vi "removeNode.vi"(0 "reference":refnum<class "AbstractNode.lvclass">, 1 "graph":refnum<class "Graph.lvclass">, 2 "node":refnum<class "AbstractNode.lvclass">, 5 "error in (no error)":errorcluster) -> (14 "reference out":refnum<class "AbstractNode.lvclass">, 19 "error out":errorcluster)   [LabVIEW 2020, in "AbstractNode.lvclass"]
uses:
  <resource>/Framework/Providers/Open_GDS/UML/AbstractNode_class/AbstractNode.lvclass
  <resource>/Framework/Providers/Open_GDS/UML/Graph_class/Graph.lvclass
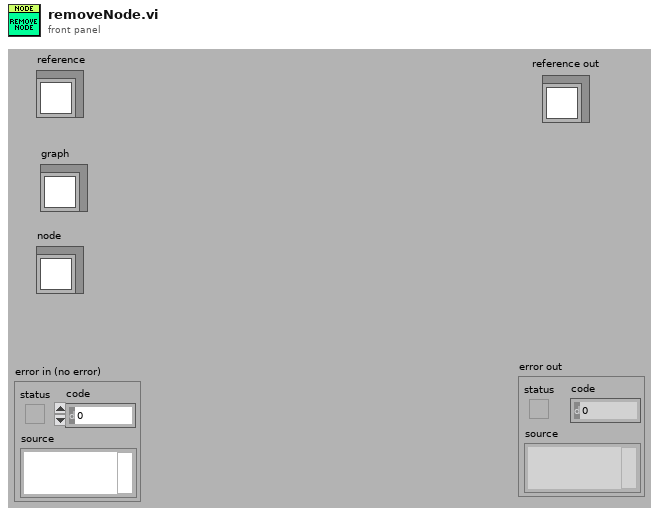
[diagram p1: front panel]
types:
  T1 = typedef "AbstractNode.lvclass/ObjectAttributes.ctl" = cluster{"parent":refnum<class "AbstractNode.lvclass">, "children":refnum<class "AbstractNode.lvclass">[], "Hidden":bool}
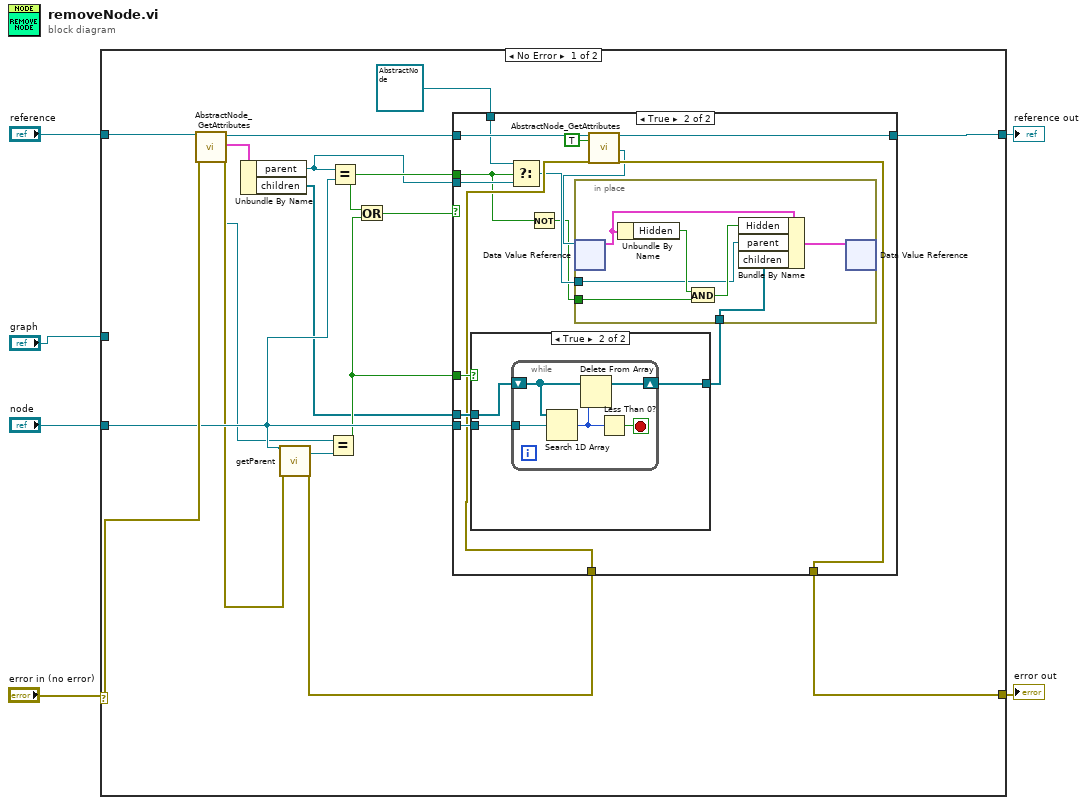
[diagram p0: block diagram]
diagram:
  n1 = case shown="No Error" "error in (no error)" {
    selector: "error in (no error)" -> [w19 w56]
    tunnel: "reference" -> [w22 w57]
    tunnel: [w21 w56] -> w5
    tunnel: [w20 w57] -> w4
    tunnel: "graph" -> [_ _]
    tunnel: "node" -> [w18 _]
    frame No Error {
      n2 = call <resource>:"AbstractNode_GetAttributes.vi"("reference in"=w22, "error in (no error)"=w19) -> ("reference out"=w9:refnum<class "AbstractNode.lvclass">, "Data"=w7:T1, "error out"=w13:errorcluster)  [unwired: 1 in, 14 out]
      n3 = Unbundle By Name(w7) -> ("parent"=w15:refnum<class "AbstractNode.lvclass">, "children"=w10:refnum<class "AbstractNode.lvclass">[])
      n4 = call-dynamic "getParent.vi"("reference"=w18, "error in (no error)"=w13) -> ("parentNode"=w12:refnum<class "AbstractNode.lvclass">, "error out"=w14:errorcluster)  [unwired: 13 in, 3 out]
      n5 = Equal?(x=w9, y=w12) -> (x = y?=w11:bool)
      n6 = Equal?(x=w15, y=w18) -> (x = y?=w16:bool)
      n7 = Or(x=w16, y=w11) -> (x .or. y?=w17:bool)
      n8 = case shown="True" w17 {
        tunnel: w9 -> [w24 w39]
        tunnel: [w24 w38] -> w20
        tunnel: w16 -> [_ w30]
        tunnel: w15 -> [_ w31]
        tunnel: w18 -> [_ w37]
        tunnel: w14 -> [w23 w33]
        tunnel: [w23 w36] -> w21
        tunnel: w11 -> [_ w35]
        tunnel: w10 -> [_ w34]
        tunnel: refnum<class "AbstractNode.lvclass"> refnum ("parent") -> [_ w32]
        frame False {
        }
        frame True {
          n9 = case shown="True" w35 {
            tunnel: w37 -> [_ w50]
            tunnel: w34 -> [w47 w49]
            tunnel: [w47 w48] -> w26
            frame False {
            }
            frame True {
              n10 = while {
                tunnel: w50 -> [w55]
                shift-right: [w53] -> w48
                shift-left: w49 -> [w54]
                stop <- w51 stop-if-true
                n11 = Search 1D Array(1D array=w54, element=w55) -> (index of element=w52:i32)  [unwired: 1 out]
                n12 = Delete From Array(array=w54, index=w52) -> (array with subset deleted=w53:refnum<class "AbstractNode.lvclass">[])  [unwired: 1 in, 1 out]
                n13 = Less Than 0?(x=w52) -> (x < 0?=w51:bool)
              }
            }
          }
          n14 = Select(t=w32, s=w30, f=w31) -> (s? t:f=w27:refnum<class "AbstractNode.lvclass">)
          n15 = Not(x=w30) -> (.not. x?=w25:bool)
          n16 = call <resource>:"AbstractNode_GetAttributes.vi"("reference in"=w39, "OnlyGetDvrReference(False)"=TRUE, "error in (no error)"=w33) -> ("reference out"=w38:refnum<class "AbstractNode.lvclass">, "DataRef"=w28:refnum<data-value>, "error out"=w36:errorcluster)  [unwired: 13 in, 1 out]
          n17 = in-place {
            in-place-border: w27 -> [w43]
            in-place-border: w26 -> [w42]
            in-place-border: w25 -> [w40]
            n18 = in-place-dvr #1(w28) -> (w46:T1)  [unwired: 1 out]
            n19 = Unbundle By Name(w46) -> ("Hidden"=w45:bool)
            n20 = And(x=w45, y=w40) -> (x .and. y?=w44:bool)
            n21 = Bundle By Name(cluster=w46, "Hidden"=w44, "parent"=w43, "children"=w42) -> (w41:T1)
            n22 = in-place-dvr #1(w41) -> ()  [unwired: 2 out]
          }
        }
      }
    }
    frame Error {
    }
  }
  "reference out" <- w4
  "error out" <- w5
